vi "XYZStage-Request speed setting command.vi"(9 "Speed to set":i32, 11 "Which speed setting command?":T1) -> (0 "Error Out (no error)":errorcluster)   [LabVIEW 2020]
uses:
  Typedefs/XYZ stage states.ctl
  Typedefs/XYZ stage data.ctl
  Typedefs/XYZ channel ring.ctl
  User Interface/Windows/Position control window/Globals/Pos ctrl window globals.vi
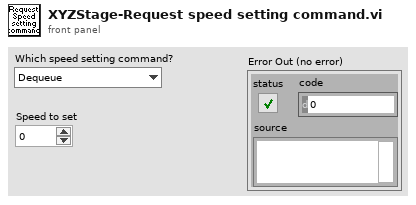
[diagram p1: front panel]
types:
  T1 = typedef "XYZ stage states.ctl" = enum16{"Dequeue", "Initialize", "Read Position", "Read Speed Setting", "Move", "Set Max Speed", "Reset Axis", "Stop all movement"}
  T2 = typedef "XYZ stage data.ctl" = cluster{"Command":T1, "Channel":T3, "X":sgl, "Y":sgl, "Z":sgl, "Speed":i32, "Zero":bool, "Use acknowledgement?":bool}
  T3 = typedef "XYZ channel ring.ctl" = string
  T4 = typedef "Pos Ctrl window refs cluster.ctl" = cluster{"menu reference":refnum<k9>, "X Coordinate ctrl":refnum<vi>, "Y Coordinate ctrl":refnum<vi>, "Z Coordinate ctrl":refnum<vi>, "Speed setting ctrl":refnum<vi>, "Up":refnum<vi>, "Down":refnum<vi>, "Left":refnum<vi>, "Right":refnum<vi>, "Z move up":refnum<vi>, "Z move down":refnum<vi>, "Down-left":refnum<vi>, "Down-right":refnum<vi>, "Up-left":refnum<vi>, "Up-right":refnum<vi>, "Step = size of image":refnum<vi>, "XY step (um)":refnum<vi>, "Z step (um)":refnum<vi>, "Speed setting\navailable":refnum<vi>}
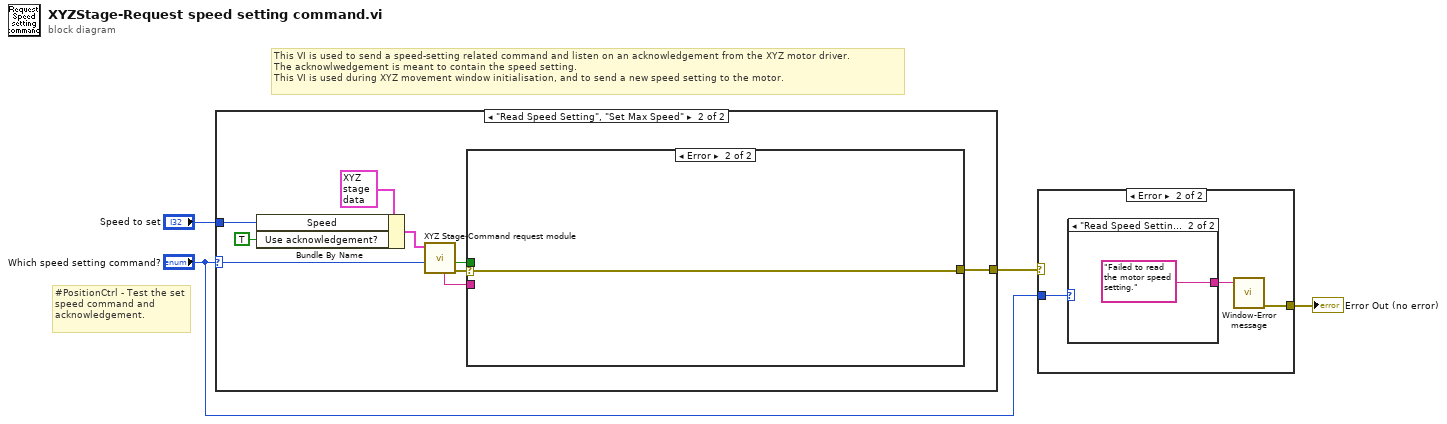
[diagram p0: block diagram]
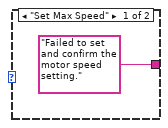
[diagram p3: hidden frame]
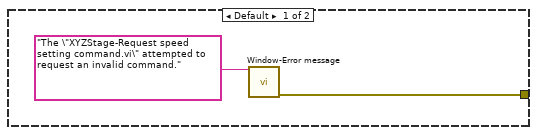
[diagram p4: hidden frame]
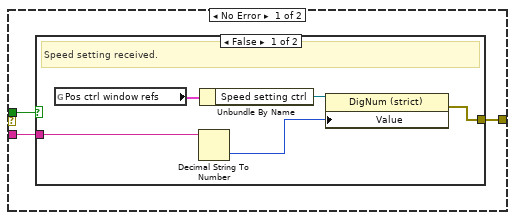
[diagram p5: hidden frame]
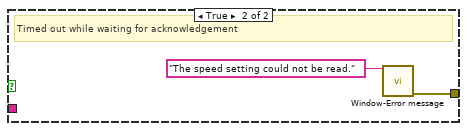
[diagram p6: hidden frame]
diagram:
  # "#PositionCtrl - Test the set speed command and acknowledgement."
  # "This VI is used to send a speed-setting related command and listen on an acknowledgement from the XYZ motor driver.\nThe acknowlwedgement is meant to contain the speed setting.\nThis VI is used during XYZ movement window initialisation, and to send a new speed setting to the motor."
  n1 = case shown="\"Read Speed Setting\", \"Set Max Speed\"" "Which speed setting command?" {
    selector: "Which speed setting command?" -> [_ w10]
    tunnel: [w5 w8] -> w3
    tunnel: "Speed to set" -> [_ w7]
    frame Default {
      n2 = call "Window-Error message.vi"("Message"="The \"XYZStage-Request speed setting command.vi\" attempted to request an invalid command." ("Error Source")) -> ("Error Out (no error)"=w5:errorcluster)  [unwired: 10 in]
    }
    frame "Read Speed Setting", "Set Max Speed" {
      n3 = Bundle By Name(cluster=T2 {"Command"=enum."Initialize", "Channel"="Z", "X"=0.0, "Y"=0.0, "Z"=0.0, "Speed"=0, "Zero"=FALSE, "Use acknowledgement?"=TRUE} ("XYZ Stage data to queue"), "Speed"=w7, "Use acknowledgement?"=TRUE ("Wait for acknowledge?")) -> (w15:T2)
      n4 = call "XYZ Stage-Command request module.vi"("Command"=w10, "XYZ Stage data to queue"=w15) -> ("error out"=w9:errorcluster, "Timed out while waiting for acknowledgement"=w11:bool, "Acknowledgement message"=w12:string)  [unwired: 5 in, 2 out]
      n5 = case shown="Error" w9 {
        selector: w9 -> [_ w26]
        tunnel: w12 -> [w18 _]
        tunnel: w11 -> [w17 _]
        tunnel: [w16 w26] -> w8
        frame No Error {
          n6 = case shown="False" w17 {
            tunnel: w18 -> [w20 _]
            tunnel: [w22 w24] -> w16
            frame False {
              # "Speed setting received."
              n7 = global read "Pos ctrl window globals.vi" "Pos ctrl window refs"() -> (w21:T4)
              n8 = Decimal String To Number(string=w20) -> (number=w19:i32)  [unwired: 2 in, 1 out]
              n9 = Unbundle By Name(w21) -> ("Speed setting ctrl"=w23:refnum<vi>)
              n10 = property on="Property Node" class="DigNum (strict)"(reference=w23, "Value"=w19) -> (error out=w22:errorcluster)  [unwired: 1 in, 1 out]
            }
            frame True {
              # "Timed out while waiting for acknowledgement"
              n11 = call "Window-Error message.vi"("Message"="The speed setting could not be read." ("Error Source")) -> ("Error Out (no error)"=w24:errorcluster)  [unwired: 10 in]
            }
          }
        }
        frame Error {
        }
      }
    }
  }
  n12 = case shown="Error" w3 {
    tunnel: "Which speed setting command?" -> [_ w29]
    tunnel: [_ w27] -> w1
    frame No Error {
    }
    frame Error {
      n13 = case shown="\"Read Speed Setting\", Default" w29 {
        tunnel: ["Failed to set and confirm the motor speed setting." "Failed to read the motor speed setting."] -> w28
        frame "Set Max Speed" {
        }
        frame "Read Speed Setting", Default {
        }
      }
      n14 = call "Window-Error message.vi"("Message"=w28) -> ("Error Out (no error)"=w27:errorcluster)  [unwired: 10 in]
    }
  }
  "Error Out (no error)" <- w1
